vi "G#Object_IsExternalCreateProcessRunning.vi"(5 "error in (no error)":errorcluster) -> (15 "external create enabled?":bool, 16 "owned by external process?":bool, 17 "external create process running?":bool, 19 "error out":errorcluster)   [LabVIEW 2020, in "G#Object.lvclass"]
doc: "Checks if external create is enabled and also if the external create process is running."
uses:
  <vilib>/addons/_AddQ/G#Object/G#Object.lvclass
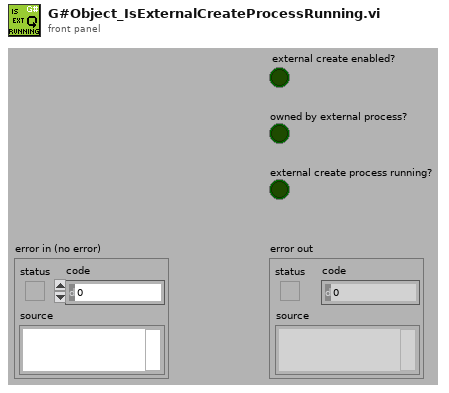
[diagram p1: front panel]
types:
  T1 = enum32{"Bad", "Idle", "Run top level", "Running"}
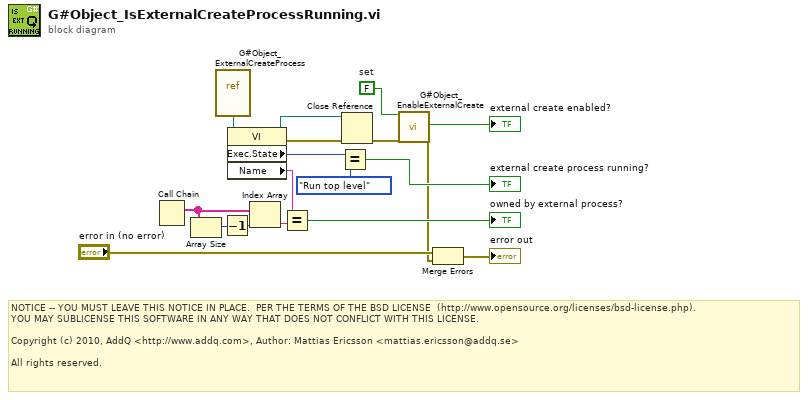
[diagram p0: block diagram]
diagram:
  w9 = FALSE  # set
  # "NOTICE -- YOU MUST LEAVE THIS NOTICE IN PLACE.  PER THE TERMS OF THE BSD LICENSE  (http://www.opensource.org/licenses/bsd-license.php).\nYOU MAY SUBLICENSE THIS SOFTWARE IN ANY WAY THAT DOES NOT CONFLICT WITH THIS LICENSE.\n\nCopyright (c) 2010, AddQ <http://www.addq.com>, Author: Mattias Ericsson <mattias.ericsson@addq.se>\n\nAll rights reserved."
  n1 = Call Chain() -> (call chain=w7:string[])
  n2 = Array Size(array=w7) -> (size(s)=w5:i32)
  n3 = vi-ref <vilib>:"G#Object_ExternalCreateProcess.vi"() -> (w15:refnum<vi>)
  n4 = Decrement(x=w5) -> (x-1=w4:i32)
  n5 = property class="VI"(reference=w15) -> (reference out=w13:refnum<vi>, error out=w14:errorcluster, "Exec.State"=w12:T1, "Name"=w8:string)  [unwired: 1 in]
  n6 = Index Array(array=w7, index=w4) -> (element=w6:string)
  n7 = Equal?(x=w8, y=w6) -> (x = y?=→"owned by external process?":bool)
  n8 = Equal?(x=w12, y=T1."Run top level" ("Execution:State")) -> (x = y?=→"external create process running?":bool)
  n9 = Close Reference(reference=w13, error in (no error)=w14) -> (error out=w10:errorcluster)
  n10 = call <vilib>:"G#Object_EnableExternalCreate.vi"("set (F)"=w9, "error in (no error)"=w10) -> ("enabled"=→"external create enabled?":bool, "error out"=w2:errorcluster)  [unwired: 15 in, 1 out]
  n11 = Merge Errors("error in (no error)", w2) -> (→"error out":errorcluster)
